vi "Actor Core.vi"(8 "error in":errorcluster, 11 "TCP_Client_Window in":refnum<class "TCP_Client_Window.lvclass">) -> (0 "error out":errorcluster, 3 "Actor out":refnum<class "Actor.lvclass">)   [LabVIEW 2023, in "TCP_Client_Window.lvlib" / "TCP_Client_Window.lvclass"]
doc: "(<B>Filename</B>: Actor Framework.lvlib:Actor.lvclass:Actor Core.vi)\n\nReceives messages to the actor, reacts to them, and initiates any error handling that may shut the actor down.\n\nDescendant classes may override this VI to append parallel tasks for the actor to complete while it handles messages. Overrides use the Call Parent Class Method node."
uses:
  TCP_Client_Window.lvclass
  <vilib>/ActorFramework/Actor/Actor.lvclass
  TCP_Server_Connection_Handler/TCP_Server_Connection_Handler/Overrides/TypeDefinitions/ControlsReferences.ctl
  TCP_Client_Window.lvclass/TCP_Client_Window.ctl
  <vilib>/ActorFramework/Actor/Actor.lvclass/Actor.ctl
  <vilib>/ActorFramework/Message Enqueuer/Message Enqueuer.lvclass/Message Enqueuer.ctl
  TCP_Client_Window Messages/SendMessageToClient Msg/SendMessageToClient Msg.lvclass/SendMessageToClient Msg.ctl
  <vilib>/ActorFramework/Message Enqueuer/Init from Existing Queue.vi
  <vilib>/ActorFramework/Message Enqueuer/Enqueue.vi
  TCP_Client_Window Messages/SendMessageToClient Msg/SendMessageToClient Msg.lvclass
  <vilib>/ActorFramework/Message Priority Queue/Priority Enqueue.vi
  <vilib>/ActorFramework/Message Enqueuer/Message Enqueuer.lvclass
  C:/Program Files (x86)/National Instruments/LabVIEW 2023/vi.lib/ActorFramework/Actor/Actor.lvclass
  C:/Source/LabVIEW/TCP_server/TCP_Client_Window/TCP_Client_Window/TCP_Client_Window.lvclass
panel:
  in  "Send Button":bool
  in  "Messages to Client":string
  out "Messages from Client":string
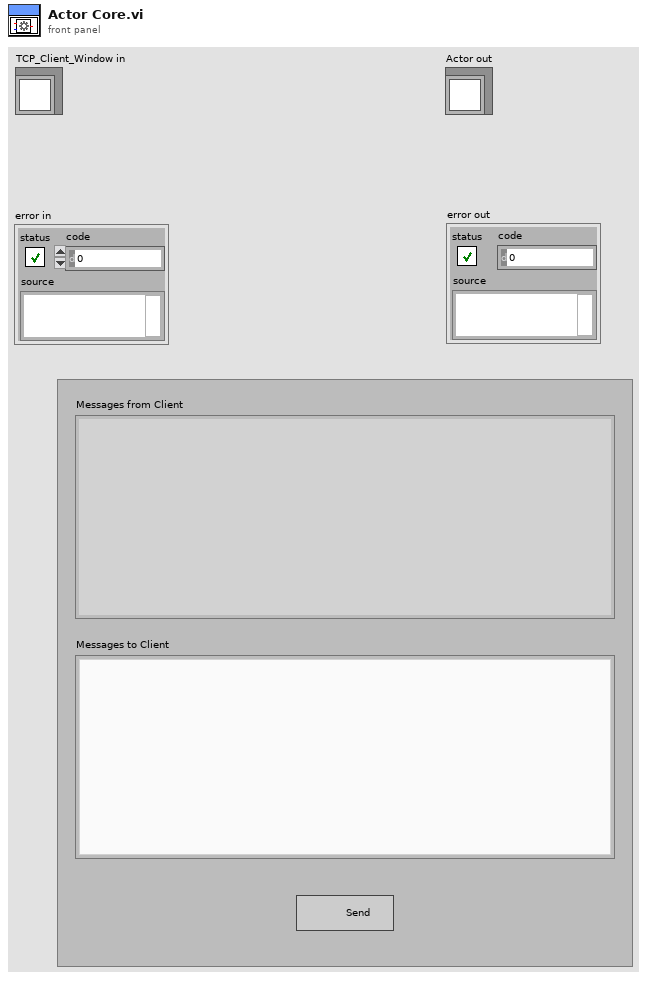
[diagram p1: front panel]
types:
  T1 = typedef "TCP_Client_Window.lvlib/TCP_Client_Window.lvclass/ControlsReferences.ctl" = cluster{"Messages from Client":refnum<vi>, "Messages to Client":refnum<vi>}
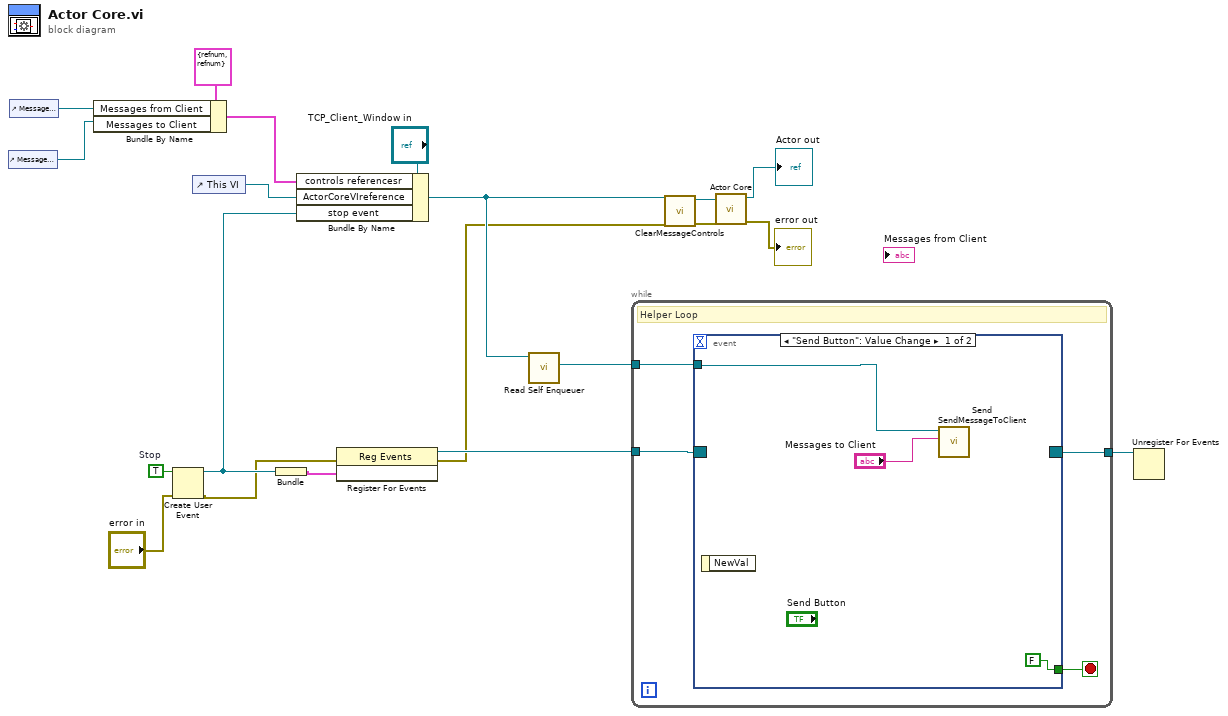
[diagram p0: block diagram]
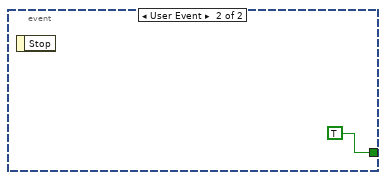
[diagram p2: hidden frame]
diagram:
  w13 = TRUE  # Stop
  n1 = control-ref of="Messages to Client"() -> (w17:refnum<vi>)
  n2 = control-ref of="Messages from Client"() -> (w18:refnum<vi>)
  n3 = Bundle By Name(cluster=T1 {"Messages from Client"=refnum, "Messages to Client"=refnum} ("output cluster"), "Messages from Client"=w18, "Messages to Client"=w17) -> (w14:T1)
  n4 = Create User Event(user event datatype=w13, error in="error in") -> (user event=w8:refnum<user-event>, error out=w7:errorcluster)
  n5 = control-ref of="This VI"() -> (w6:refnum<vi>)
  n6 = Bundle("Stop"=w8) -> (w12:cluster{"Stop":refnum<user-event>})  [unwired: 1 in]
  n7 = Bundle By Name(cluster="TCP_Client_Window in", "controls referencesr"=w14, "ActorCoreVIreference"=w6, "stop event"=w8) -> (w4:refnum<class "TCP_Client_Window.lvclass">)
  n8 = register-events(error in=w7, w12) -> (reference out=w11:refnum<event-registration>, error out=w3:errorcluster)  [unwired: 1 in]
  n9 = call <vilib>:"Read Self Enqueuer.vi"("Actor"=w4) -> ("Self Enqueuer"=w9:refnum<class "Message Enqueuer.lvclass">)  [unwired: 10 in]
  n10 = while {
    tunnel: w11 -> [w23]
    tunnel: [w22] -> w10
    tunnel: w9 -> [w21]
    stop <- w24 stop-if-true
    # "Helper Loop"
    n11 = event shown="[0] \"Send Button\": Value Change" {
      selector: w23 -> [_ _]
      dyn-events: [_ _] -> w22
      timeout: _ -> [_ _]
      tunnel: [FALSE TRUE] -> w24
      tunnel: w21 -> [w26 _]
      event "Send Button": Value Change {
        n12 = event-data() -> ()  [unwired: 1 in, 1 out]
        n13 = call "Send SendMessageToClient.vi"("Message"="Messages to Client", "Message Enqueuer"=w26) -> ()  [unwired: 8 in, 2 out]
      }
      event User Event {
        n14 = event-data() -> ()  [unwired: 1 in, 1 out]
      }
    }
  }
  n15 = call "ClearMessageControls.vi"("error in (no error)"=w3, "TCP_Client_Window in"=w4) -> ("error out"=w2:errorcluster, "TCP_Client_Window out"=w1:refnum<class "TCP_Client_Window.lvclass">)  [unwired: 8 in]
  n16 = call-parent "Actor Core.vi"("error in"=w2, "Actor in"=w1) -> ("error out"=→"error out":errorcluster, "Actor out"=→"Actor out":refnum<class "Actor.lvclass">)  [unwired: 8 in]
  n17 = Unregister For Events(event registration refnum=w10) -> ()  [unwired: 1 in, 1 out]
